vi "SigProc_method scriptFGV.vi"(5 "Function":enum16{"Read", "Write", "Init"}(ring)=enum."Write", 6 "error in":errorcluster, 8 "Script in":string, 9 "dup path":path) -> (0 "error out":errorcluster, 2 "Script out":string)   [LabVIEW 2018, in "Sig2MS.lvclass"]
uses:
  Sig2MS.lvclass
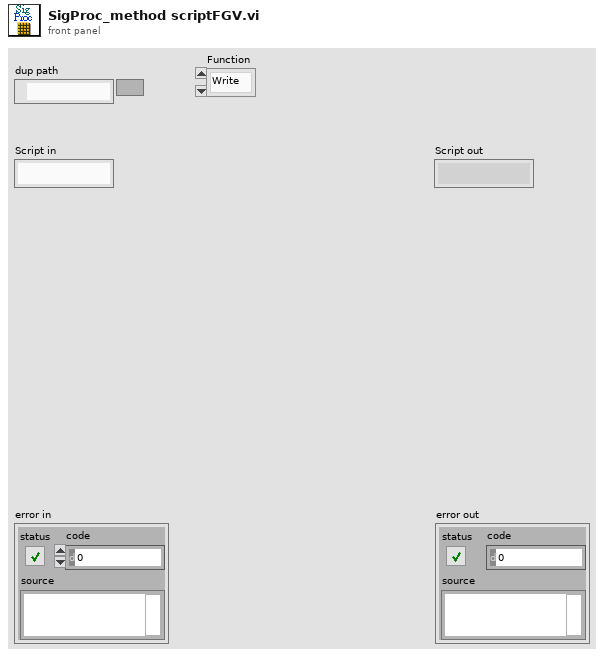
[diagram p1: front panel]
types:
  T1 = enum16{"open", "replace", "create", "open or create", "replace or create", "replace or create with confirmation"}
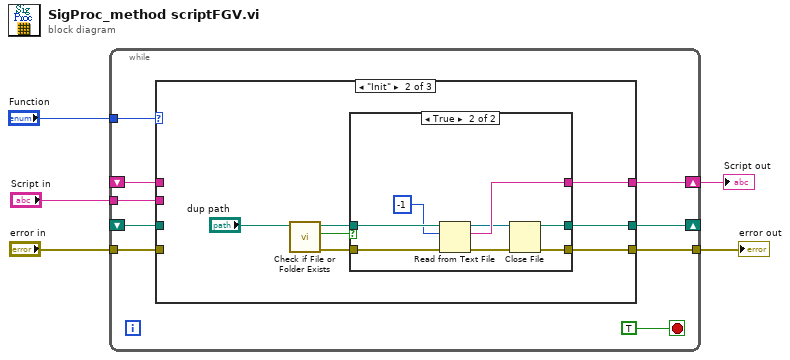
[diagram p0: block diagram]
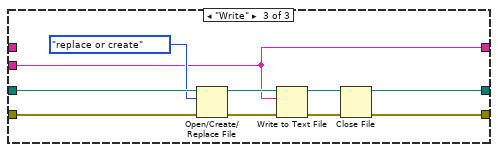
[diagram p4: hidden frame]
diagram:
  n1 = while {
    tunnel: "Function" -> [w14]
    shift-right: [w12] -> w3
    shift-left: _ -> [w10]
    tunnel: "Script in" -> [w11]
    shift-right: [w9] -> _
    shift-left: _ -> [w8]
    tunnel: "error in" -> [w7]
    tunnel: [w6] -> w1
    stop <- TRUE stop-if-true
    n2 = case shown="\"Init\"" w14 {
      tunnel: w11 -> [_ _ w38]
      tunnel: [w17 w24 w38] -> w12
      tunnel: w10 -> [w17 _ _]
      tunnel: [w16 w23 w37] -> w9
      tunnel: w8 -> [w16 _ w44]
      tunnel: w7 -> [w15 _ w36]
      tunnel: [w15 w22 w35] -> w6
      frame "Read", Default {
      }
      frame "Init" {
        n3 = call <vilib>:"Check if File or Folder Exists.vi"("path"="dup path") -> ("error out"=w18:errorcluster, "file or folder exists?"=w19:bool, "dup path"=w20:path)  [unwired: 8 in]
        n4 = case shown="True" w19 {
          tunnel: w20 -> [w26 w34]
          tunnel: w18 -> [w25 w33]
          tunnel: [_ w32] -> w24
          tunnel: [w26 w28] -> w23
          tunnel: [w25 w27] -> w22
          frame False {
          }
          frame True {
            n5 = Read from Text File(file (use dialog)=w34, count=-1, error in=w33) -> (refnum out=w29:refnum<file>, text=w32:string, error out=w30:errorcluster)  [unwired: 1 in, 1 out]
            n6 = Close File(refnum=w29, error in=w30) -> (path=w28:path, error out=w27:errorcluster)
          }
        }
      }
      frame "Write" {
        n7 = Open/Create/Replace File(file path (use dialog)=w44, error in=w36, operation (0:open)=T1."replace or create") -> (refnum out=w42:refnum<file>, error out=w40:errorcluster)  [unwired: 3 in, 1 out]
        n8 = Write to Text File(file (use dialog)=w42, text=w38, error in=w40) -> (refnum out=w41:refnum<file>, error out=w39:errorcluster)  [unwired: 1 in, 1 out]
        n9 = Close File(refnum=w41, error in=w39) -> (path=w37:path, error out=w35:errorcluster)
      }
    }
  }
  "Script out" <- w3
  "error out" <- w1
